vi "SetParameter.vi"(8 "error in (no error)":errorcluster, 10 "SetParameter":T1, 11 "NHRDCPowerModel in":refnum<class "NHRDCPowerModel.lvclass">) -> (0 "error out":errorcluster, 2 "StatusUpdates":string[](array[string]), 3 "NHRDCPowerModel out":refnum<class "NHRDCPowerModel.lvclass">)   [LabVIEW 2018, in "AcPwrPlugins.lvlib" / "NHRDCPowerModel.lvclass"]
uses:
  NHRDCPowerModel.lvclass
  AcPwrBaseClass/TypeDefs/SetParameterInputs.ctl
  AcPwrBaseClass/AcPwrBase.lvclass
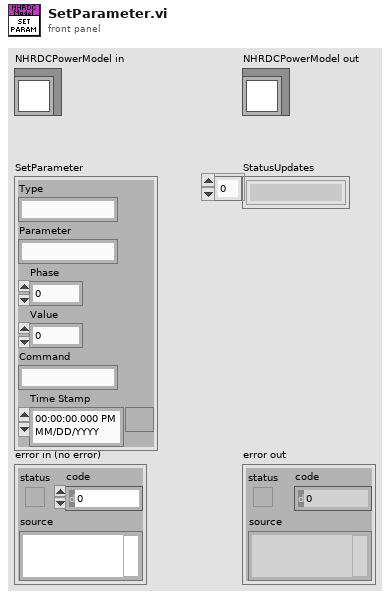
[diagram p1: front panel]
types:
  T1 = typedef "AcPwrPlugins.lvlib/AcPwrBase.lvclass/SetParameterInputs.ctl" = cluster{"Type":string, "Parameter":string, "Phase":i32, "Value":dbl, "Command":string, "Time Stamp":timestamp}
  T2 = cluster{"Voltage (V)":dbl, "Current (A)":dbl, "Resistance (Ohm)":dbl, "Power (W)":dbl, "btnV_Enable":bool, "btnI_enable":bool, "btnR_enable":bool, "btnP_enable":bool}
  T3 = typedef "AcPwrPlugins.lvlib/NHRDCPower.lvclass/Measurements.ctl" = cluster{"Handle":string, "Name":string, "Enabled":bool, "Measurement Value":sgl, "Measurement Type":enum16{"Power", "Current", "Voltage"}}[]
  T4 = typedef "AcPwrPlugins.lvlib/NHRDCPower.lvclass/Device(s)Settings.ctl" = cluster{"MeasName":string, "Modules":T5}
  T5 = typedef "AcPwrPlugins.lvlib/NHRDCPower.lvclass/Modules.ctl" = cluster{"Handle":string, "Name":string, "id query (Yes)":bool, "reset device (Yes)":bool, "Connected":bool, "Initial Battery Detect Voltage (0)":dbl, "SafetySettings":cluster{"SetWatchDog?":bool, "Voltage (V)":dbl, "Current (A)":dbl, "Power (W)":dbl, "Voltage Delay (s)":dbl, "Current Delay (s)":dbl, "Power Delay (s)":dbl}, "Options String":string, "Aperture Time (s)":dbl, "operating state (Off)":i32, "OutputSettings":cluster{"Voltage (V)":dbl, "Current (A)":dbl, "Resistance (Ohms)":dbl, "Power (W)":dbl, "Enable Voltage":bool, "Enable Current":bool, "Enable Resistance":bool, "Enable Power":bool, "Macro After Step Delay  (s)":dbl, "Wait Value (V, A, W)":dbl, "Enable Wait":bool, "Wait on Value":i32}, "SlewRate":cluster{"Set Voltage Rate V/S":dbl, "Set Current Rate A/S":dbl, "Set Resistance Rate R/S":dbl, "Set Power Rate W/S":dbl}, "Macro":cluster{"Save Macro?":bool, "Load Macro From File?":bool, "Run Macro Continuously?":bool, "Use Macros?":bool, "Load Macro File Path":path, "Save Macro File Path":string}, "Regulation Gain (1=100%)":dbl, "UpdatingOntheFly":bool}[]
  T6 = typedef "AcPwrShared.lvlib/Database Settings.ctl" = cluster{"Data Source":string, "ICDAS to Model Table":string, "Model to ICDAS Table":string}
  T7 = cluster{"Handle":string, "Name":string, "id query (Yes)":bool, "reset device (Yes)":bool, "Connected":bool, "Initial Battery Detect Voltage (0)":dbl, "SafetySettings":cluster{"SetWatchDog?":bool, "Voltage (V)":dbl, "Current (A)":dbl, "Power (W)":dbl, "Voltage Delay (s)":dbl, "Current Delay (s)":dbl, "Power Delay (s)":dbl}, "Options String":string, "Aperture Time (s)":dbl, "operating state (Off)":i32, "OutputSettings":cluster{"Voltage (V)":dbl, "Current (A)":dbl, "Resistance (Ohms)":dbl, "Power (W)":dbl, "Enable Voltage":bool, "Enable Current":bool, "Enable Resistance":bool, "Enable Power":bool, "Macro After Step Delay  (s)":dbl, "Wait Value (V, A, W)":dbl, "Enable Wait":bool, "Wait on Value":i32}, "SlewRate":cluster{"Set Voltage Rate V/S":dbl, "Set Current Rate A/S":dbl, "Set Resistance Rate R/S":dbl, "Set Power Rate W/S":dbl}, "Macro":cluster{"Save Macro?":bool, "Load Macro From File?":bool, "Run Macro Continuously?":bool, "Use Macros?":bool, "Load Macro File Path":path, "Save Macro File Path":string}, "Regulation Gain (1=100%)":dbl, "UpdatingOntheFly":bool}
  T8 = cluster{"Handle":string, "Name":string, "id query (Yes)":bool, "reset device (Yes)":bool, "Connected":bool, "Initial Battery Detect Voltage (0)":dbl, "SafetySettings":cluster{"SetWatchDog?":bool, "Voltage (V)":dbl, "Current (A)":dbl, "Power (W)":dbl, "Voltage Delay (s)":dbl, "Current Delay (s)":dbl, "Power Delay (s)":dbl}, "Options String":string, "Aperture Time (s)":dbl, "operating state (Off)":i32, "OutputSettings":cluster{"Voltage (V)":dbl, "Current (A)":dbl, "Resistance (Ohms)":dbl, "Power (W)":dbl, "Enable Voltage":bool, "Enable Current":bool, "Enable Resistance":bool, "Enable Power":bool, "Macro After Step Delay  (s)":dbl, "Wait Value (V, A, W)":dbl, "Enable Wait":bool, "Wait on Value":i32}, "SlewRate":cluster{"Set Voltage Rate V/S":dbl, "Set Current Rate A/S":dbl, "Set Resistance Rate R/S":dbl, "Set Power Rate W/S":dbl}, "Macro":cluster{"Save Macro?":bool, "Load Macro From File?":bool, "Run Macro Continuously?":bool, "Use Macros?":bool, "Load Macro File Path":path, "Save Macro File Path":string}, "Regulation Gain (1=100%)":dbl, "UpdatingOntheFly":bool}[]
  T9 = cluster{"Voltage (V)":dbl, "Current (A)":dbl, "Resistance (Ohms)":dbl, "Power (W)":dbl, "Enable Voltage":bool, "Enable Current":bool, "Enable Resistance":bool, "Enable Power":bool, "Macro After Step Delay  (s)":dbl, "Wait Value (V, A, W)":dbl, "Enable Wait":bool, "Wait on Value":i32}
  T10 = cluster{"Device(s)Settings":T4, "Database Settings":T6}
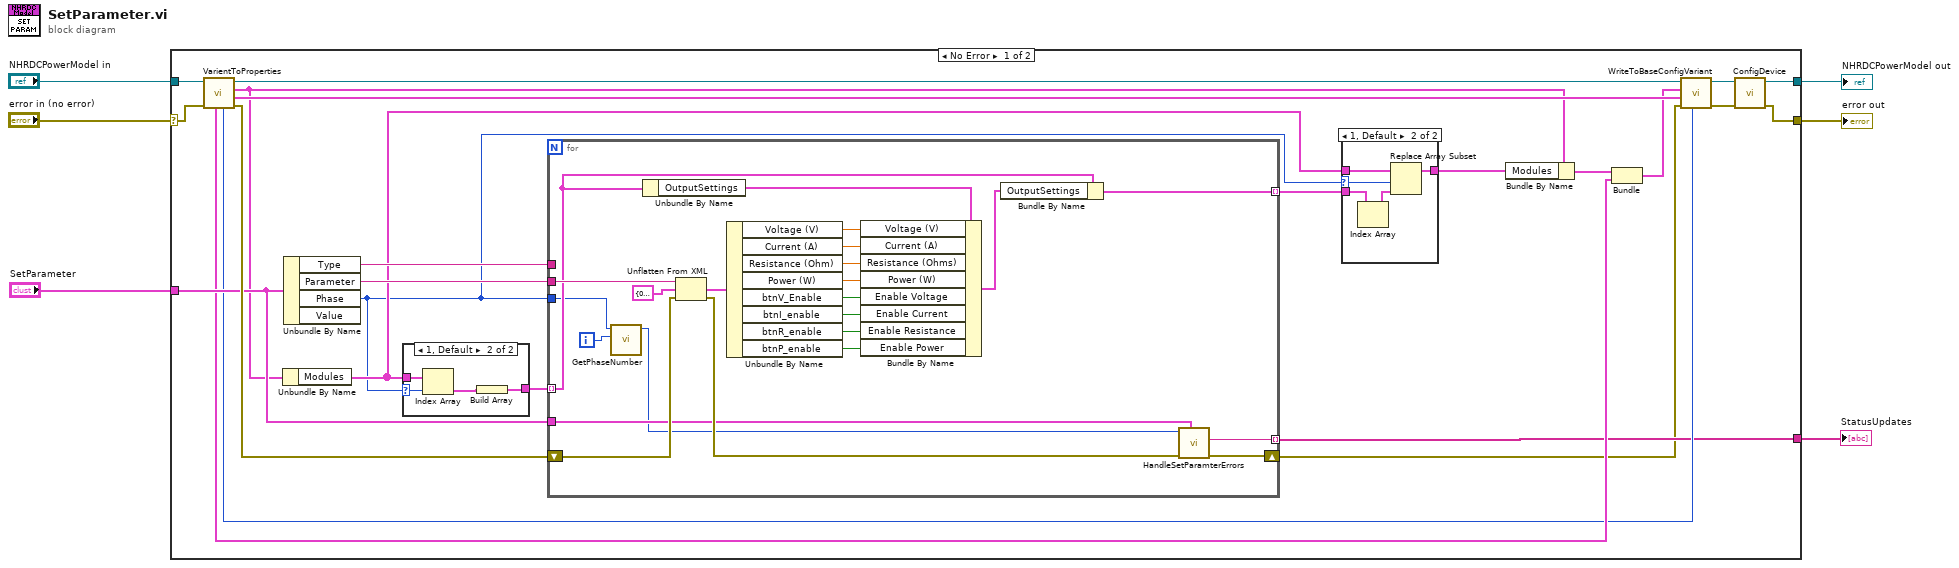
[diagram p0: block diagram]
diagram:
  n1 = case shown="No Error" "error in (no error)" {
    selector: "error in (no error)" -> [w29 w66]
    tunnel: [w8 w66] -> w5
    tunnel: "NHRDCPowerModel in" -> [w30 w65]
    tunnel: [w9 w65] -> w3
    tunnel: "SetParameter" -> [w21 _]
    tunnel: [w13 _] -> w1
    frame No Error {
      n2 = call "VarientToProperties.vi"("error in (no error)"=w29, "AcPwrPlugins.lvlib:NHRDCModel.lvclass"=w30) -> ("error out"=w23:errorcluster, "Measurements"=w24:T3, "Device(s)Settings"=w19:T4, "AcPwrPlugins.lvlib:NHRDCModel.lvclass"=w25:refnum<class "NHRDCPowerModel.lvclass">, "Measurement Refresh Time (ms)"=w15:u32, "Database Settings"=w16:T6)  [unwired: 4 in]
      n3 = Unbundle By Name(w19) -> ("Modules"=w22:T5)
      n4 = Unbundle By Name(w21) -> ("Type"=w27:string, "Parameter"=w26:string, "Phase"=w7:i32)  [unwired: 1 out]
      n5 = case shown="1, Default" w7 {
        selector: w7 -> [_ w64]
        tunnel: w22 -> [w60 w63]
        tunnel: [w60 w61] -> w28
        frame -1 {
        }
        frame 1, Default {
          n6 = Index Array(array=w63, index=w64) -> (element=w62:T7)
          n7 = Build Array(w62) -> (w61:T8)
        }
      }
      n8 = for {
        tunnel: w28 -> [w46] mode=indexing
        tunnel: w7 -> [w42]
        tunnel: w27 -> [_]
        tunnel: w26 -> [w59]
        shift-right: [w39] -> w12
        shift-left: w23 -> [w57]
        tunnel: w21 -> [w43]
        tunnel: [w38] -> w20 mode=indexing
        tunnel: [w37] -> w13 mode=indexing
        i -> [w41]
        n9 = call "GetPhaseNumber.vi"("Loop Counter"=w41, "Phase(-1, all) in"=w42) -> ("Phase(-1, all) out"=w40:i32)  [unwired: 9 in]
        n10 = Unbundle By Name(w46) -> ("OutputSettings"=w47:T9)
        n11 = Unflatten From XML(xml string=w59, type=T2 {"Voltage (V)"=0.0, "Current (A)"=0.0, "Resistance (Ohm)"=0.0, "Power (W)"=0.0, "btnV_Enable"=FALSE, "btnI_enable"=FALSE, "btnR_enable"=FALSE, "btnP_enable"=FALSE} ("output cluster"), error in (no error)=w57) -> (value=w56:T2, error out=w44:errorcluster)
        n12 = Unbundle By Name(w56) -> ("Voltage (V)"=w48:dbl, "Current (A)"=w49:dbl, "Resistance (Ohm)"=w50:dbl, "Power (W)"=w51:dbl, "btnV_Enable"=w52:bool, "btnI_enable"=w53:bool, "btnR_enable"=w54:bool, "btnP_enable"=w55:bool)
        n13 = Bundle By Name(cluster=w47, "Voltage (V)"=w48, "Current (A)"=w49, "Resistance (Ohms)"=w50, "Power (W)"=w51, "Enable Voltage"=w52, "Enable Current"=w53, "Enable Resistance"=w54, "Enable Power"=w55) -> (w45:T9)
        n14 = Bundle By Name(cluster=w46, "OutputSettings"=w45) -> (w38:T7)
        n15 = call "HandleSetParamterErrors.vi"("SetParameter"=w43, "error in (no error)"=w44, "Phase"=w40) -> ("error IO"=w39:errorcluster, "Status Update"=w37:string)  [unwired: 7 in]
      }
      n16 = case shown="1, Default" w7 {
        selector: w7 -> [_ w35]
        tunnel: w22 -> [_ w36]
        tunnel: w20 -> [w31 w34]
        tunnel: [w31 w32] -> w18
        frame -1 {
        }
        frame 1, Default {
          n17 = Index Array(array=w34) -> (element=w33:T7)  [unwired: 1 in]
          n18 = Replace Array Subset(array=w36, new element=w33, index=w35) -> (w32:T5)
        }
      }
      n19 = Bundle By Name(cluster=w19, "Modules"=w18) -> (w17:T4)
      n20 = Bundle("Device(s)Settings"=w17, "Database Settings"=w16) -> (w14:T10)  [unwired: 1 in]
      n21 = call-dynamic "WriteToBaseConfigVariant.vi"("Measurement Refresh Time (ms)"=w15, "error in (no error)"=w12, "Meas"=w24, "Config"=w14, "NHRDCModel in"=w25) -> ("error out"=w11:errorcluster, "NHRDCModel out"=w10:refnum<class "NHRDCPowerModel.lvclass">)  [unwired: 5 in]
      n22 = call-dynamic "ConfigDevice.vi"("error in (no error)"=w11, "NHRDCModel in"=w10) -> ("error out"=w8:errorcluster, "NHRDCModel out"=w9:refnum<class "NHRDCPowerModel.lvclass">)  [unwired: 8 in]
    }
    frame Error {
    }
  }
  "error out" <- w5
  "NHRDCPowerModel out" <- w3
  "StatusUpdates" <- w1
